vi "Setup camera parameters.vi"(8 "error in (no error)":errorcluster, 11 "Retiga in":refnum<class "Retiga.lvclass">) -> (0 "error out":errorcluster, 3 "Retiga out":refnum<class "Retiga.lvclass">)   [LabVIEW 2012, in "Retiga.lvclass"]
uses:
  Retiga.lvclass
  Retiga.lvclass/Retiga.ctl
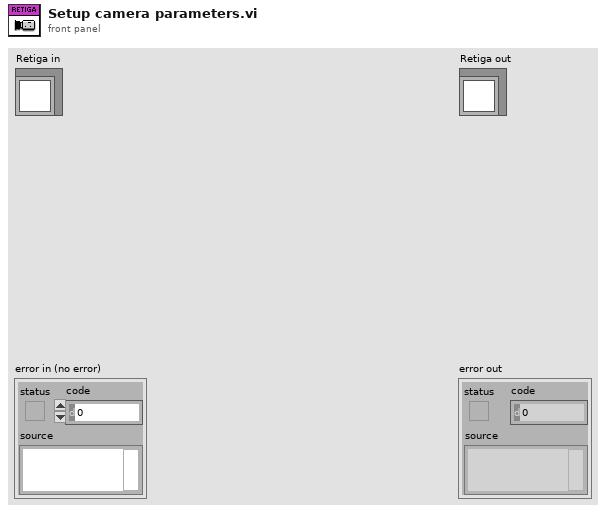
[diagram p1: front panel]
types:
  T1 = enum32{"gain", "offset", "exposure", "binning", "horizontal binning", "vertical binning", "readout speed", "trigger type", "lcd filter", "cooler", "exposure red", "exposure blue", "image format", "roi x", "roi y", "roi width", "roi height", "reserved1", "shutter state", "reserved2", "sync-b out", "reserved3", "intensifier gain", "trigger delay", "camera mode", "normalized gain", "normalized intenifier gain DB", "doPostProcessing", "postProcessGainRed", "postProcessGainGreen", "postProcessGainBlue", "postProcessBayerAlgorithm", "postProcessImageFormat", "fan", "blackout mode", "high sensitivity", "Readout Port", "EM Gain", "open delay", "close delay", "clearing mode"}
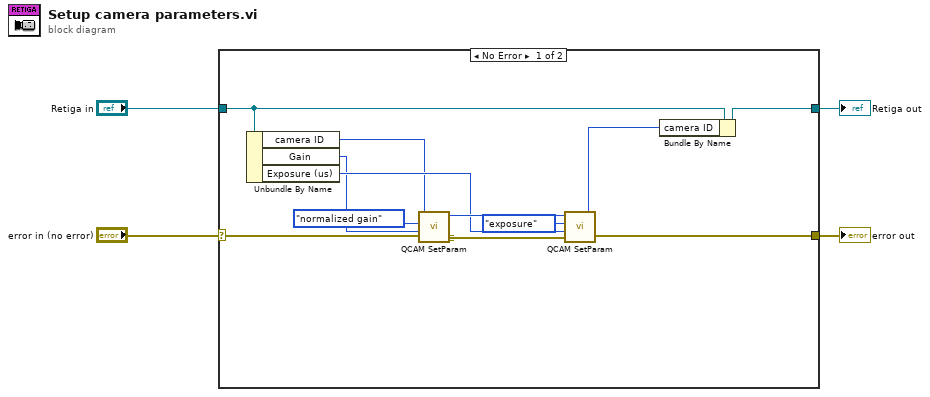
[diagram p0: block diagram]
diagram:
  n1 = case shown="No Error" "error in (no error)" {
    selector: "error in (no error)" -> [w12 w18]
    tunnel: [w11 w18] -> w3
    tunnel: [w9 w17] -> w1
    tunnel: "Retiga in" -> [w10 w17]
    frame No Error {
      n2 = Unbundle By Name(w10) -> ("camera ID"=w6:u32, "Gain"=w5:i32, "Exposure (us)"=w7:i32)
      n3 = call <userlib>:"QCAM SetParam.vi"("error in (no error)"=w12, "value"=w5, "parameter key"=T1."normalized gain", "cameraId"=w6) -> ("error out"=w14:errorcluster, "cameraId out"=w15:u32)
      n4 = call <userlib>:"QCAM SetParam.vi"("error in (no error)"=w14, "value"=w7, "parameter key"=T1."exposure", "cameraId"=w15) -> ("error out"=w11:errorcluster, "cameraId out"=w8:u32)
      n5 = Bundle By Name(cluster=w10, "camera ID"=w8) -> (w9:refnum<class "Retiga.lvclass">)
    }
    frame Error {
    }
  }
  "error out" <- w3
  "Retiga out" <- w1
